vi "DAQ.vi"() -> (0 "Error Out":errorcluster)   [LabVIEW 2017]
uses:
  <vilib>/dex/Flush And Wait Empty Condition.ctl
  <vilib>/Platform/TimedLoop/XDataNode/timing_clust.ctl
  <vilib>/Platform/TimedLoop/XDataNode/nitl_modes.ctl
  <vilib>/Platform/TimedLoop/XDataNode/wakeup.ctl
  <vilib>/DAQmx/read.llb/DAQmx Read (Analog 1D DBL NChan 1Samp).vi
  <vilib>/DAQmx/miscellaneous.llb/DAQmx Fill In Error Info.vi
  <vilib>/Platform/TimedLoop/XDataNode/XDataNode.xnode
  <vilib>/Platform/TimedLoop/XDataNode/XDNodeRunTimeDep.lvlib
  <resource>/objmgr/ni.dex.rc
panel:
  out "Producer Loop Time":i64
  out "Consumer Loop Time":u32
  in  "Error In":errorcluster
  out "Time":dbl
  out "Available Elements for Writing":i32
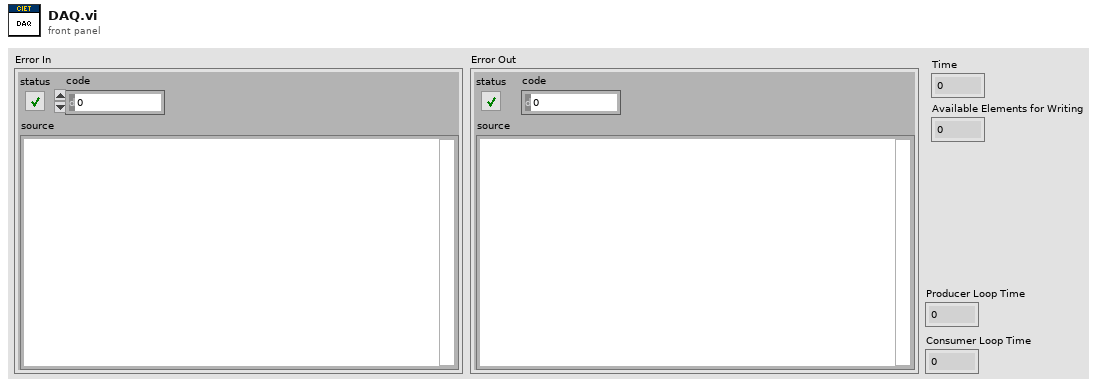
[diagram p1: front panel]
types:
  T1 = typedef "Flush And Wait Empty Condition.ctl" = u8
  T2 = typedef "XDNodeRunTimeDep.lvlib/timing_clust.ctl" = cluster{"Expected End [f-1]":u64, "Actual End [f-1]":u64, "Finished Late? [f-1]":bool, "Expected End [i-1]":u64, "Actual End [i-1]":u64, "Finished Late? [i-1]":bool, "Expected Start [i]":u64, "Actual Start [i]":u64, "Expected Start [f]":u64, "Actual Start [f]":u64, "Source Name":string, "Structure Name":string, "Period":i64, "Deadline":i64, "Offset":i64, "Start":i64, "Priority":i32, "Timeout":i32, "Mode":T3, "Wakeup Reason":T4, "Error":errorcluster, "Source Type":string, "Secondary Source Type":string, "Global End Time":u64, "Global Start Time":u64, "Frame Duration":u64, "Iteration Duration":u64, "Assigned CPU":i32, "I/O Scan Engine Mode":u32}
  T3 = typedef "XDNodeRunTimeDep.lvlib/nitl_modes.ctl" = enum32{"No Change", "Process missed periods, maintain original phase", "Discard missed periods, maintain original phase", "Process missed periods, ignore original phase", "Discard missed periods, ignore original phase"}
  T4 = typedef "XDNodeRunTimeDep.lvlib/wakeup.ctl" = enum32{"Normal", "Aborted", "Asynchronous wakeup", "Timing source error", "Timed loop error", "Timeout"}
  T5 = cluster{"[0]":sgl, "[1]":sgl, "[2]":sgl, "[3]":sgl, "[4]":sgl, "[5]":sgl, "[6]":sgl, "[7]":sgl, "[8]":sgl, "[9]":sgl, "[10]":sgl, "[11]":sgl, "[12]":sgl, "[13]":sgl, "[14]":sgl, "[15]":sgl, "[16]":sgl, "[17]":sgl, "[18]":sgl, "[19]":sgl, "[20]":sgl, "[21]":sgl, "[22]":sgl, "[23]":sgl, "[24]":sgl, "[25]":sgl, "[26]":sgl, "[27]":sgl, "[28]":sgl, "[29]":sgl, "[30]":sgl, "[31]":sgl, "[32]":sgl, "[33]":sgl, "[34]":sgl, "[35]":sgl, "[36]":sgl, "[37]":sgl, "[38]":sgl, "[39]":sgl, "[40]":sgl, "[41]":sgl, "[42]":sgl, "[43]":sgl, "[44]":sgl, "[45]":sgl, "[46]":sgl, "[47]":sgl, "[48]":sgl, "[49]":sgl, "[50]":sgl, "[51]":sgl, "[52]":sgl, "[53]":sgl, "[54]":sgl, "[55]":sgl, "[56]":sgl}
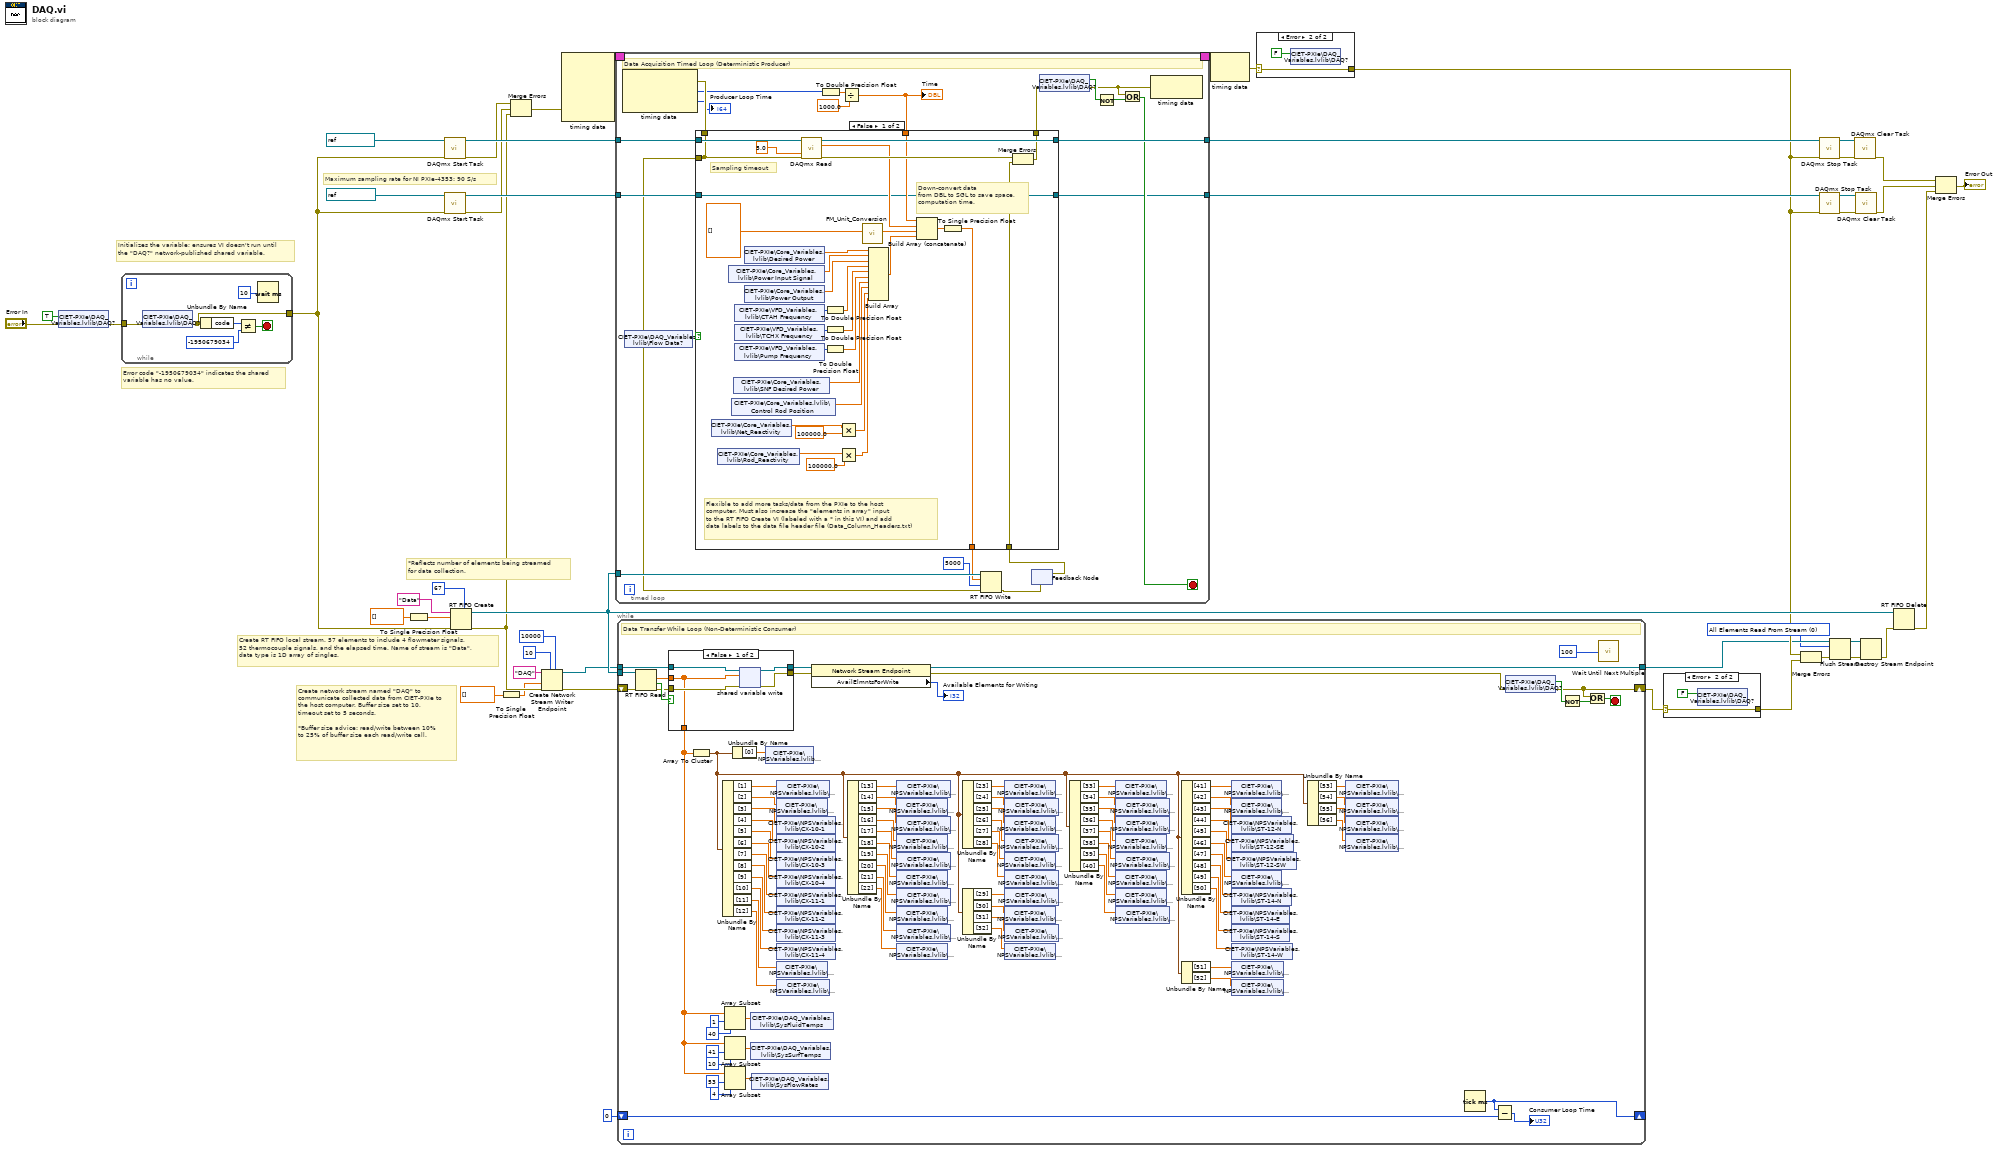
[diagram p0: block diagram]
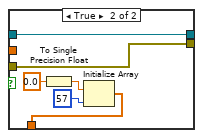
[diagram p4: hidden frame]
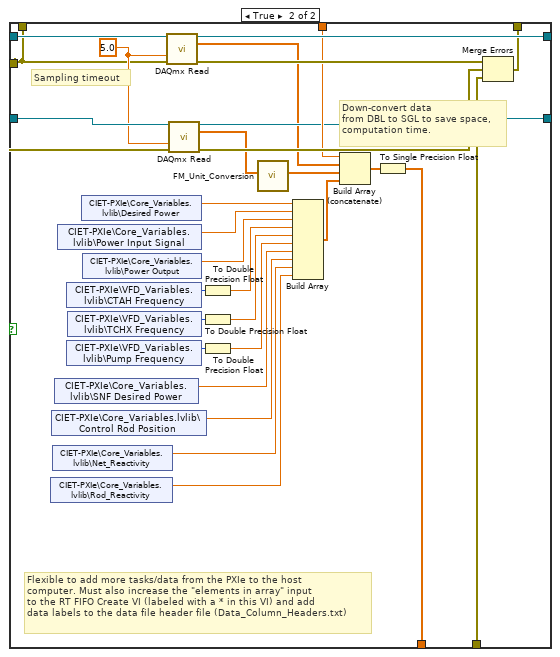
[diagram p5: hidden frame]
diagram:
  w3 = T1 0 items=["All Elements Read From Stream", "All Elements Available for Reading"] ("wait condition")
  # "*Reflects number of elements being streamed\nfor data collection."
  # "Create RT FIFO local stream. 57 elements to include 4 flowmeter signals,\n52 thermocouple signals, and the elapsed time. Name of stream is \"Data\",\ndata type is 1D array of singles."
  # "Create network stream named \"DAQ\" to communicate collected data from CIET-PXIe to the host computer. Buffer size set to 10, timeout set to 5 seconds. \n\n*Buffer size advice: read/write between 10%\nto 25% of buffer size each read/write call."
  # "Maximum sampling rate for NI PXIe-4353: 90 S/s"
  # "Initializes the variable; ensures VI doesn't run until\nthe \"DAQ?\" network-published shared variable."
  # "Error code \"-1950679034\" indicates the shared\nvariable has no value."
  n1 = shared-variable "CIET-PXIe\\DAQ_Variables.lvlib\\DAQ?"(TRUE ("Active?"), error in="Error In") -> (error out=w23:errorcluster)
  n2 = while {
    tunnel: w23 -> [w52]
    tunnel: [w51] -> w22
    stop <- w48 stop-if-true
    n3 = shared-variable "CIET-PXIe\\DAQ_Variables.lvlib\\DAQ?"(error in=w52) -> (error out=w51:errorcluster)  [unwired: 1 out]
    n4 = Unbundle By Name(w51) -> ("code"=w50:i32)
    n5 = Not Equal?(x=w50, y=-1950679034) -> (x != y?=w48:bool)
    n6 = Wait (ms)(milliseconds to wait=u32 10) -> ()  [unwired: 1 out]
  }
  n7 = To Single Precision Float(number=dbl[] []) -> (single precision float=w33:sgl[])
  n8 = call <vilib>:"DAQmx Start Task.vi"("task/channels in"=refnum<k21> "CIET-TC", "error in"=w22) -> ("task out"=w43:refnum<k21>, "error out"=w27:errorcluster)  [unwired: 12 in]
  n9 = call <vilib>:"DAQmx Start Task.vi"("task/channels in"=refnum<k21> "CIET-FM", "error in"=w22) -> ("task out"=w42:refnum<k21>, "error out"=w28:errorcluster)  [unwired: 12 in]
  n10 = RT FIFO Create(0:"Data" ("name (unnamed)"), 1:w33, 3:w22, 6:u32 67 ("elements in array (1)")) -> (8:w26:refnum<k33>, 11:w18:errorcluster)  [unwired: 4 in, 1 out]
  n11 = To Single Precision Float(number=dbl[] []) -> (single precision float=w8:sgl[])
  n12 = Merge Errors(w27, w28, w18) -> (w29:errorcluster)
  n13 = Create Network Stream Writer Endpoint(5:10000 ("timeout in ms (-1)"), 7:10 ("writer buffer size"), 8:w18, 9:w8, 11:"DAQ" ("writer name")) -> (0:w19:errorcluster, 3:w17:refnum<k21>)  [unwired: 2 in]
  n14 = node-c288(w29) -> (w47:T2)  [unwired: 4 in]
  n15 = timed-loop {
    timing: w47 -> [_]
    timing-out: [_] -> w46
    tunnel: w26 -> [w72]
    tunnel: w43 -> [w75]
    tunnel: [w73] -> w37
    tunnel: w42 -> [w74]
    tunnel: [w60] -> w36
    stop <- w67 stop-if-true
    # "Data Acquisition Timed Loop (Deterministic Producer)"
    n16 = node-c288() -> (w70:errorcluster, w61:i64, →"Producer Loop Time":i64)  [unwired: 1 in]
    n17 = shared-variable "CIET-PXIe\\DAQ_Variables.lvlib\\Flow Data?"() -> (w55:bool)  [unwired: 1 in, 1 out]
    n18 = To Double Precision Float(number=w61) -> (double precision float=w64:dbl)
    n19 = Divide(x=w64, y=1000.0) -> (x/y=w63:dbl)
    "Time" <- w63
    n20 = feedback #1() -> (w56:errorcluster)  [unwired: 1 in]
    n21 = case shown="False" w55 {
      tunnel: w75 -> [w107 w137]
      tunnel: w74 -> [w87 w136]
      tunnel: [w105 w134] -> w73
      tunnel: [w103 w132] -> w58
      tunnel: w70 -> [w84 w112]
      tunnel: w56 -> [w85 w129]
      tunnel: [w101 w128] -> w66
      tunnel: w63 -> [w100 w127]
      tunnel: [w87 w126] -> w60
      tunnel: [w84 w112] -> w54
      frame False {
        # "Flexible to add more tasks/data from the PXIe to the host \ncomputer. Must also increase the \"elements in array\" input \nto the RT FIFO Create VI (labeled with a * in this VI) and add\ndata labels to the data file header file (Data_Column_Headers.txt)"
        # "Down-convert data\nfrom DBL to SGL to save space,\ncomputation time."
        # "Sampling timeout"
        n22 = shared-variable "CIET-PXIe\\Core_Variables.lvlib\\Net_Reactivity"() -> (w76:dbl)  [unwired: 1 in, 1 out]
        n23 = shared-variable "CIET-PXIe\\Core_Variables.lvlib\\Rod_Reactivity"() -> (w80:dbl)  [unwired: 1 in, 1 out]
        n24 = shared-variable "CIET-PXIe\\Core_Variables.lvlib\\Power Input Signal"() -> (w90:dbl)  [unwired: 1 in, 1 out]
        n25 = shared-variable "CIET-PXIe\\Core_Variables.lvlib\\Control Rod Position"() -> (w82:dbl)  [unwired: 1 in, 1 out]
        n26 = shared-variable "CIET-PXIe\\Core_Variables.lvlib\\SNF Desired Power"() -> (w83:dbl)  [unwired: 1 in, 1 out]
        n27 = shared-variable "CIET-PXIe\\VFD_Variables.lvlib\\CTAH Frequency"() -> (w92:u16)  [unwired: 1 in, 1 out]
        n28 = shared-variable "CIET-PXIe\\VFD_Variables.lvlib\\Pump Frequency"() -> (w94:u16)  [unwired: 1 in, 1 out]
        n29 = shared-variable "CIET-PXIe\\VFD_Variables.lvlib\\TCHX Frequency"() -> (w93:u16)  [unwired: 1 in, 1 out]
        n30 = shared-variable "CIET-PXIe\\Core_Variables.lvlib\\Desired Power"() -> (w89:dbl)  [unwired: 1 in, 1 out]
        n31 = shared-variable "CIET-PXIe\\Core_Variables.lvlib\\Power Output"() -> (w91:dbl)  [unwired: 1 in, 1 out]
        n32 = call-poly <vilib>:"DAQmx Read.vi"("task/channels in"=w107, "timeout"=5.0, "error in"=w84) -> ("task out"=w105:refnum<k21>, "data"=w99:dbl[], "error out"=w102:errorcluster)  [unwired: 10 in]
        n33 = To Double Precision Float(number=w92) -> (double precision float=w95:dbl)
        n34 = To Double Precision Float(number=w93) -> (double precision float=w96:dbl)
        n35 = To Double Precision Float(number=w94) -> (double precision float=w97:dbl)
        n36 = Multiply(x=w76, y=100000.0) -> (x*y=w77:dbl)
        n37 = Multiply(x=w80, y=100000.0) -> (x*y=w81:dbl)
        n38 = call "FM_Unit_Conversion.vi"("Input Array [A]"=dbl[] []) -> ("Output Array [kg/h]"=w98:dbl[])  [unwired: 10 in]
        n39 = Build Array(w89, w90, w91, w95, w96, w97, w83, w82, w77, w81) -> (w88:dbl[])
        n40 = Build Array (concatenate)(w100, w99, w98, w88) -> (w104:dbl[])
        n41 = To Single Precision Float(number=w104) -> (single precision float=w103:sgl[])
        n42 = Merge Errors(w102, w85) -> (w101:errorcluster)
      }
      frame True {
        w135 = 5.0 ("timeout")
        # "Flexible to add more tasks/data from the PXIe to the host \ncomputer. Must also increase the \"elements in array\" input \nto the RT FIFO Create VI (labeled with a * in this VI) and add\ndata labels to the data file header file (Data_Column_Headers.txt)"
        # "Down-convert data\nfrom DBL to SGL to save space,\ncomputation time."
        # "Sampling timeout"
        n43 = shared-variable "CIET-PXIe\\Core_Variables.lvlib\\Rod_Reactivity"() -> (w108:dbl)  [unwired: 1 in, 1 out]
        n44 = shared-variable "CIET-PXIe\\Core_Variables.lvlib\\Control Rod Position"() -> (w110:dbl)  [unwired: 1 in, 1 out]
        n45 = shared-variable "CIET-PXIe\\Core_Variables.lvlib\\Net_Reactivity"() -> (w109:dbl)  [unwired: 1 in, 1 out]
        n46 = shared-variable "CIET-PXIe\\Core_Variables.lvlib\\SNF Desired Power"() -> (w111:dbl)  [unwired: 1 in, 1 out]
        n47 = shared-variable "CIET-PXIe\\Core_Variables.lvlib\\Power Input Signal"() -> (w115:dbl)  [unwired: 1 in, 1 out]
        n48 = shared-variable "CIET-PXIe\\VFD_Variables.lvlib\\CTAH Frequency"() -> (w117:u16)  [unwired: 1 in, 1 out]
        n49 = shared-variable "CIET-PXIe\\VFD_Variables.lvlib\\Pump Frequency"() -> (w119:u16)  [unwired: 1 in, 1 out]
        n50 = shared-variable "CIET-PXIe\\VFD_Variables.lvlib\\TCHX Frequency"() -> (w118:u16)  [unwired: 1 in, 1 out]
        n51 = shared-variable "CIET-PXIe\\Core_Variables.lvlib\\Desired Power"() -> (w114:dbl)  [unwired: 1 in, 1 out]
        n52 = shared-variable "CIET-PXIe\\Core_Variables.lvlib\\Power Output"() -> (w116:dbl)  [unwired: 1 in, 1 out]
        n53 = call-poly <vilib>:"DAQmx Read.vi"("task/channels in"=w137, "timeout"=w135, "error in"=w112) -> ("task out"=w134:refnum<k21>, "data"=w125:dbl[], "error out"=w130:errorcluster)  [unwired: 10 in]
        n54 = call-poly <vilib>:"DAQmx Read.vi"("task/channels in"=w136, "timeout"=w135, "error in"=w112) -> ("task out"=w126:refnum<k21>, "data"=w123:dbl[], "error out"=w131:errorcluster)  [unwired: 10 in]
        n55 = To Double Precision Float(number=w117) -> (double precision float=w120:dbl)
        n56 = To Double Precision Float(number=w118) -> (double precision float=w121:dbl)
        n57 = To Double Precision Float(number=w119) -> (double precision float=w122:dbl)
        n58 = call "FM_Unit_Conversion.vi"("Input Array [A]"=w123) -> ("Output Array [kg/h]"=w124:dbl[])  [unwired: 10 in]
        n59 = Build Array(w114, w115, w116, w120, w121, w122, w111, w110, w109, w108) -> (w113:dbl[])
        n60 = Build Array (concatenate)(w127, w125, w124, w113) -> (w133:dbl[])
        n61 = To Single Precision Float(number=w133) -> (single precision float=w132:sgl[])
        n62 = Merge Errors(w130, w131, w129) -> (w128:errorcluster)
      }
    }
    n63 = RT FIFO Write(0:w72, 1:w58, 2:5000 ("timeout in ms (0)"), 3:w54) -> (11:w57:errorcluster)  [unwired: 1 in, 3 out]
    n64 = feedback-in #1(w57) -> ()
    n65 = shared-variable "CIET-PXIe\\DAQ_Variables.lvlib\\DAQ?"(error in=w66) -> (w69:bool, error out=w65:errorcluster)
    n66 = Not(x=w69) -> (.not. x?=w68:bool)
    n67 = Or(x=w65, y=w68) -> (x .or. y?=w67:bool)
    n68 = node-c288(w65) -> ()  [unwired: 1 out]
  }
  n69 = while {
    tunnel: w26 -> [w231]
    shift-right: [w220] -> w20
    shift-left: w19 -> [w230]
    tunnel: w17 -> [w222]
    tunnel: [w217] -> w10
    shift-right: [w157] -> _
    shift-left: u32 0 ("millisecond timer value") -> [w156]
    stop <- w223 stop-if-true
    # "Data Transfer While Loop (Non-Deterministic Consumer)"
    n70 = RT FIFO Read(0:w231, 3:w230) -> (9:w227:sgl[], 10:w228:bool, 11:w226:errorcluster)  [unwired: 2 in, 2 out]
    n71 = case shown="False" w228 {
      tunnel: w227 -> [w232 _]
      tunnel: w226 -> [w236 w242]
      tunnel: [w235 w242] -> w219
      tunnel: w222 -> [w234 w241]
      tunnel: [w233 w241] -> w218
      tunnel: [w232 w237] -> w148
      frame False {
        n72 = shared-variable-write(w234, w236, w232) -> (w233:refnum<k21>, w235:errorcluster)  [unwired: 1 in, 1 out]
      }
      frame True {
        n73 = To Single Precision Float(number=sgl 0.0) -> (single precision float=w240:sgl)
        n74 = Initialize Array(w240, 57 ("dimension size")) -> (w237:sgl[])
      }
    }
    n75 = Array To Cluster(array=w148) -> (cluster=w158:T5)
    n76 = Unbundle By Name(w158) -> ("[1]"=w214:sgl, "[2]"=w213:sgl, "[3]"=w212:sgl, "[4]"=w211:sgl, "[5]"=w210:sgl, "[6]"=w209:sgl, "[7]"=w208:sgl, "[8]"=w207:sgl, "[9]"=w206:sgl, "[10]"=w205:sgl, "[11]"=w204:sgl, "[12]"=w203:sgl)
    n77 = Array Subset(array=w148, index=1, length=40) -> (w152:sgl[])
    n78 = Array Subset(array=w148, index=41, length=10) -> (w150:sgl[])
    n79 = Array Subset(array=w148, index=53, length=4) -> (w145:sgl[])
    n80 = Unbundle By Name(w158) -> ("[0]"=w215:sgl)
    n81 = shared-variable "CIET-PXIe\\DAQ_Variables.lvlib\\SysFluidTemps"(w152) -> ()  [unwired: 1 in, 1 out]
    n82 = shared-variable "CIET-PXIe\\DAQ_Variables.lvlib\\SysSurfTemps"(w150) -> ()  [unwired: 1 in, 1 out]
    n83 = shared-variable "CIET-PXIe\\DAQ_Variables.lvlib\\SysFlowRates"(w145) -> ()  [unwired: 1 in, 1 out]
    n84 = shared-variable "CIET-PXIe\\NPSVariables.lvlib\\Time"(w215) -> ()  [unwired: 1 in, 1 out]
    n85 = shared-variable "CIET-PXIe\\NPSVariables.lvlib\\WT-10"(w214) -> ()  [unwired: 1 in, 1 out]
    n86 = shared-variable "CIET-PXIe\\NPSVariables.lvlib\\BT-11"(w213) -> ()  [unwired: 1 in, 1 out]
    n87 = shared-variable "CIET-PXIe\\NPSVariables.lvlib\\CX-10-1"(w212) -> ()  [unwired: 1 in, 1 out]
    n88 = shared-variable "CIET-PXIe\\NPSVariables.lvlib\\CX-10-2"(w211) -> ()  [unwired: 1 in, 1 out]
    n89 = shared-variable "CIET-PXIe\\NPSVariables.lvlib\\CX-10-3"(w210) -> ()  [unwired: 1 in, 1 out]
    n90 = shared-variable "CIET-PXIe\\NPSVariables.lvlib\\CX-10-4"(w209) -> ()  [unwired: 1 in, 1 out]
    n91 = shared-variable "CIET-PXIe\\NPSVariables.lvlib\\CX-11-1"(w208) -> ()  [unwired: 1 in, 1 out]
    n92 = shared-variable "CIET-PXIe\\NPSVariables.lvlib\\CX-11-2"(w207) -> ()  [unwired: 1 in, 1 out]
    n93 = shared-variable "CIET-PXIe\\NPSVariables.lvlib\\CX-11-3"(w206) -> ()  [unwired: 1 in, 1 out]
    n94 = shared-variable "CIET-PXIe\\NPSVariables.lvlib\\CX-11-4"(w205) -> ()  [unwired: 1 in, 1 out]
    n95 = shared-variable "CIET-PXIe\\NPSVariables.lvlib\\BT-12"(w204) -> ()  [unwired: 1 in, 1 out]
    n96 = shared-variable "CIET-PXIe\\NPSVariables.lvlib\\WT-13"(w203) -> ()  [unwired: 1 in, 1 out]
    n97 = property class="Network Stream Endpoint"(reference=w218, error in=w219) -> (reference out=w217:refnum<k21>, error out=w216:errorcluster, "AvailElmntsForWrite"=→"Available Elements for Writing":i32)
    n98 = Unbundle By Name(w158) -> ("[13]"=w202:sgl, "[14]"=w201:sgl, "[15]"=w200:sgl, "[16]"=w199:sgl, "[17]"=w198:sgl, "[18]"=w197:sgl, "[19]"=w196:sgl, "[20]"=w195:sgl, "[21]"=w194:sgl, "[22]"=w193:sgl)
    n99 = shared-variable "CIET-PXIe\\NPSVariables.lvlib\\WT-20"(w202) -> ()  [unwired: 1 in, 1 out]
    n100 = shared-variable "CIET-PXIe\\NPSVariables.lvlib\\BT-21"(w201) -> ()  [unwired: 1 in, 1 out]
    n101 = shared-variable "CIET-PXIe\\NPSVariables.lvlib\\WT-22"(w200) -> ()  [unwired: 1 in, 1 out]
    n102 = shared-variable "CIET-PXIe\\NPSVariables.lvlib\\BT-23"(w199) -> ()  [unwired: 1 in, 1 out]
    n103 = shared-variable "CIET-PXIe\\NPSVariables.lvlib\\WT-24"(w198) -> ()  [unwired: 1 in, 1 out]
    n104 = shared-variable "CIET-PXIe\\NPSVariables.lvlib\\BT-25"(w197) -> ()  [unwired: 1 in, 1 out]
    n105 = shared-variable "CIET-PXIe\\NPSVariables.lvlib\\WT-26"(w196) -> ()  [unwired: 1 in, 1 out]
    n106 = shared-variable "CIET-PXIe\\NPSVariables.lvlib\\BT-27"(w195) -> ()  [unwired: 1 in, 1 out]
    n107 = shared-variable "CIET-PXIe\\NPSVariables.lvlib\\WT-28"(w194) -> ()  [unwired: 1 in, 1 out]
    n108 = shared-variable "CIET-PXIe\\NPSVariables.lvlib\\BT-29"(w193) -> ()  [unwired: 1 in, 1 out]
    n109 = Unbundle By Name(w158) -> ("[23]"=w192:sgl, "[24]"=w191:sgl, "[25]"=w190:sgl, "[26]"=w189:sgl, "[27]"=w188:sgl, "[28]"=w187:sgl)
    n110 = Unbundle By Name(w158) -> ("[29]"=w186:sgl, "[30]"=w185:sgl, "[31]"=w184:sgl, "[32]"=w183:sgl)
    n111 = shared-variable "CIET-PXIe\\NPSVariables.lvlib\\BT-30"(w192) -> ()  [unwired: 1 in, 1 out]
    n112 = shared-variable "CIET-PXIe\\NPSVariables.lvlib\\WT-31"(w191) -> ()  [unwired: 1 in, 1 out]
    n113 = shared-variable "CIET-PXIe\\NPSVariables.lvlib\\BT-32"(w190) -> ()  [unwired: 1 in, 1 out]
    n114 = shared-variable "CIET-PXIe\\NPSVariables.lvlib\\WT-33"(w189) -> ()  [unwired: 1 in, 1 out]
    n115 = shared-variable "CIET-PXIe\\NPSVariables.lvlib\\BT-34"(w188) -> ()  [unwired: 1 in, 1 out]
    n116 = shared-variable "CIET-PXIe\\NPSVariables.lvlib\\WT-35"(w187) -> ()  [unwired: 1 in, 1 out]
    n117 = shared-variable "CIET-PXIe\\NPSVariables.lvlib\\WT-40"(w186) -> ()  [unwired: 1 in, 1 out]
    n118 = shared-variable "CIET-PXIe\\NPSVariables.lvlib\\BT-41"(w185) -> ()  [unwired: 1 in, 1 out]
    n119 = shared-variable "CIET-PXIe\\NPSVariables.lvlib\\WT-42"(w184) -> ()  [unwired: 1 in, 1 out]
    n120 = shared-variable "CIET-PXIe\\NPSVariables.lvlib\\BT-43"(w183) -> ()  [unwired: 1 in, 1 out]
    n121 = Unbundle By Name(w158) -> ("[33]"=w182:sgl, "[34]"=w181:sgl, "[35]"=w180:sgl, "[36]"=w179:sgl, "[37]"=w178:sgl, "[38]"=w177:sgl, "[39]"=w176:sgl, "[40]"=w175:sgl)
    n122 = shared-variable "CIET-PXIe\\NPSVariables.lvlib\\BT-60"(w182) -> ()  [unwired: 1 in, 1 out]
    n123 = shared-variable "CIET-PXIe\\NPSVariables.lvlib\\WT-61"(w181) -> ()  [unwired: 1 in, 1 out]
    n124 = shared-variable "CIET-PXIe\\NPSVariables.lvlib\\WT-62"(w180) -> ()  [unwired: 1 in, 1 out]
    n125 = shared-variable "CIET-PXIe\\NPSVariables.lvlib\\BT-63"(w179) -> ()  [unwired: 1 in, 1 out]
    n126 = shared-variable "CIET-PXIe\\NPSVariables.lvlib\\WT-64"(w178) -> ()  [unwired: 1 in, 1 out]
    n127 = shared-variable "CIET-PXIe\\NPSVariables.lvlib\\BT-65"(w177) -> ()  [unwired: 1 in, 1 out]
    n128 = shared-variable "CIET-PXIe\\NPSVariables.lvlib\\BT-66"(w176) -> ()  [unwired: 1 in, 1 out]
    n129 = shared-variable "CIET-PXIe\\NPSVariables.lvlib\\WT-67"(w175) -> ()  [unwired: 1 in, 1 out]
    n130 = Unbundle By Name(w158) -> ("[41]"=w174:sgl, "[42]"=w173:sgl, "[43]"=w172:sgl, "[44]"=w171:sgl, "[45]"=w170:sgl, "[46]"=w169:sgl, "[47]"=w168:sgl, "[48]"=w167:sgl, "[49]"=w166:sgl, "[50]"=w165:sgl)
    n131 = Unbundle By Name(w158) -> ("[51]"=w164:sgl, "[52]"=w163:sgl)
    n132 = shared-variable "CIET-PXIe\\NPSVariables.lvlib\\ST-10"(w174) -> ()  [unwired: 1 in, 1 out]
    n133 = shared-variable "CIET-PXIe\\NPSVariables.lvlib\\ST-11"(w173) -> ()  [unwired: 1 in, 1 out]
    n134 = shared-variable "CIET-PXIe\\NPSVariables.lvlib\\ST-12-N"(w172) -> ()  [unwired: 1 in, 1 out]
    n135 = shared-variable "CIET-PXIe\\NPSVariables.lvlib\\ST-12-SE"(w171) -> ()  [unwired: 1 in, 1 out]
    n136 = shared-variable "CIET-PXIe\\NPSVariables.lvlib\\ST-12-SW"(w170) -> ()  [unwired: 1 in, 1 out]
    n137 = shared-variable "CIET-PXIe\\NPSVariables.lvlib\\ST-13"(w169) -> ()  [unwired: 1 in, 1 out]
    n138 = shared-variable "CIET-PXIe\\NPSVariables.lvlib\\ST-14-N"(w168) -> ()  [unwired: 1 in, 1 out]
    n139 = shared-variable "CIET-PXIe\\NPSVariables.lvlib\\ST-14-E"(w167) -> ()  [unwired: 1 in, 1 out]
    n140 = shared-variable "CIET-PXIe\\NPSVariables.lvlib\\ST-14-S"(w166) -> ()  [unwired: 1 in, 1 out]
    n141 = shared-variable "CIET-PXIe\\NPSVariables.lvlib\\ST-14-W"(w165) -> ()  [unwired: 1 in, 1 out]
    n142 = shared-variable "CIET-PXIe\\NPSVariables.lvlib\\AT-01"(w164) -> ()  [unwired: 1 in, 1 out]
    n143 = shared-variable "CIET-PXIe\\NPSVariables.lvlib\\AT-02"(w163) -> ()  [unwired: 1 in, 1 out]
    n144 = Unbundle By Name(w158) -> ("[53]"=w162:sgl, "[54]"=w161:sgl, "[55]"=w160:sgl, "[56]"=w159:sgl)
    n145 = shared-variable "CIET-PXIe\\NPSVariables.lvlib\\FM-20"(w162) -> ()  [unwired: 1 in, 1 out]
    n146 = shared-variable "CIET-PXIe\\NPSVariables.lvlib\\FM-30"(w161) -> ()  [unwired: 1 in, 1 out]
    n147 = shared-variable "CIET-PXIe\\NPSVariables.lvlib\\FM-40"(w160) -> ()  [unwired: 1 in, 1 out]
    n148 = shared-variable "CIET-PXIe\\NPSVariables.lvlib\\FM-60"(w159) -> ()  [unwired: 1 in, 1 out]
    n149 = Tick Count (ms)() -> (millisecond timer value=w157:u32)
    n150 = Subtract(x=w157, y=w156) -> (x-y=→"Consumer Loop Time":u32)
    n151 = shared-variable "CIET-PXIe\\DAQ_Variables.lvlib\\DAQ?"(error in=w216) -> (w225:bool, error out=w220:errorcluster)
    n152 = Not(x=w225) -> (.not. x?=w224:bool)
    n153 = Or(x=w220, y=w224) -> (x .or. y?=w223:bool)
    n154 = call "Wait Until Next Multiple"("Count(mSec)"=u32 100) -> ()  [unwired: 1 out]
  }
  n155 = node-c288(w46) -> (w21:errorcluster)
  n156 = case shown="Error" w21 {
    selector: w21 -> [w243 w244]
    tunnel: [w243 w244] -> w16
    frame No Error {
    }
    frame Error {
      n157 = shared-variable "CIET-PXIe\\DAQ_Variables.lvlib\\DAQ?"(FALSE ("DAQ?")) -> ()  [unwired: 1 in, 1 out]
    }
  }
  n158 = case shown="Error" w20 {
    selector: w20 -> [w246 w247]
    tunnel: [w246 w247] -> w15
    frame No Error {
    }
    frame Error {
      n159 = shared-variable "CIET-PXIe\\DAQ_Variables.lvlib\\DAQ?"(FALSE ("DAQ?")) -> ()  [unwired: 1 in, 1 out]
    }
  }
  n160 = Merge Errors(w16, w15) -> (w12:errorcluster)
  n161 = call <vilib>:"DAQmx Stop Task.vi"("task/channels in"=w37, "error in"=w16) -> ("task out"=w40:refnum<k21>, "error out"=w41:errorcluster)  [unwired: 12 in]
  n162 = call <vilib>:"DAQmx Stop Task.vi"("task/channels in"=w36, "error in"=w16) -> ("task out"=w38:refnum<k21>, "error out"=w39:errorcluster)  [unwired: 12 in]
  n163 = Flush Stream(8:w12, 10:w3, 11:w10) -> (0:w14:errorcluster, 3:w13:refnum<k21>)  [unwired: 1 in, 1 out]
  n164 = call <vilib>:"DAQmx Clear Task.vi"("task in"=w40, "error in"=w41) -> ("error out"=w35:errorcluster)  [unwired: 13 in]
  n165 = call <vilib>:"DAQmx Clear Task.vi"("task in"=w38, "error in"=w39) -> ("error out"=w34:errorcluster)  [unwired: 13 in]
  n166 = Destroy Stream Endpoint(8:w14, 11:w13) -> (0:w11:errorcluster)
  n167 = RT FIFO Delete(0:w26, 3:w11) -> (11:w5:errorcluster)  [unwired: 1 in]
  n168 = Merge Errors(w35, w34, w5) -> (→"Error Out":errorcluster)
